vi "GFITS_LibOpenImage.vi"(8 "error in (no error)":errorcluster, 11 "imname":string="/home/bonati/images/chiron/test.fits") -> (0 "error out":errorcluster, 2 "return value":u64, 3 "imname out":string)   [LabVIEW 2016]
uses:
  c/lib/libgfits.so
panel:
  in  "err":i32
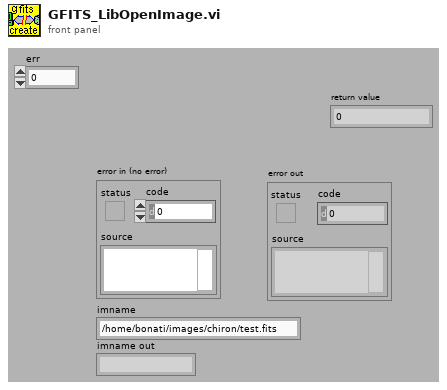
[diagram p1: front panel]
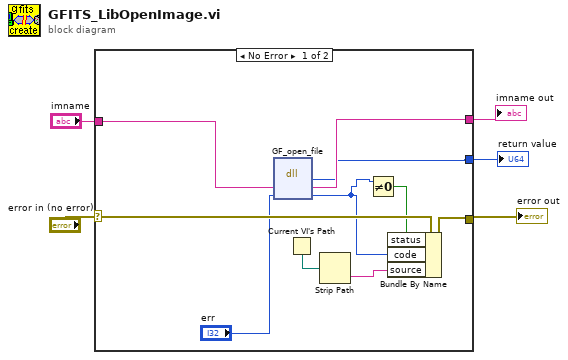
[diagram p0: block diagram]
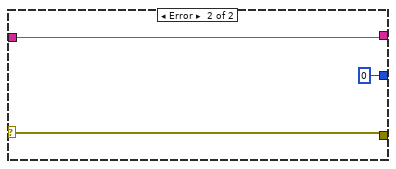
[diagram p2: hidden frame]
diagram:
  n1 = case shown="No Error" "error in (no error)" {
    selector: "error in (no error)" -> [w15 w18]
    tunnel: [w6 0] -> w5
    tunnel: [w11 w18] -> w3
    tunnel: "imname" -> [w10 w16]
    tunnel: [w9 w16] -> w1
    frame No Error {
      n2 = dll-call lib="home/simager/panview/PAN/Modules/GFITS/private/c/lib/libgfits.so" fn="GF_open_file"("imname"=w10, "err"="err") -> ("return type"=w6:u64, "imname"=w9:string, "err"=w7:i32)  [unwired: 3 in, 2 out]
      n3 = Current VI's Path() -> (path=w13:path)
      n4 = Strip Path(path=w13) -> (name=w12:string)  [unwired: 1 out]
      n5 = Not Equal To 0?(x=w7) -> (x != 0?=w14:bool)
      n6 = Bundle By Name(cluster=w15, "status"=w14, "code"=w7, "source"=w12) -> (w11:errorcluster)
    }
    frame Error {
    }
  }
  "return value" <- w5
  "error out" <- w3
  "imname out" <- w1
